vi "分层图显示1.2.1（看别的）.vi"(11 "IN":string) -> (3 "OUT":string)   [LabVIEW 2016]
uses:
  <vilib>/Utility/file.llb/Read Delimited Spreadsheet (DBL).vi
  <vilib>/Utility/file.llb/Read Delimited Spreadsheet (I64).vi
panel:
  in  "更换色码":bool
  in  "色码表导入":path=path "C:/Users/H301/Desktop/art闭环扫描程序/色码表/色码表（彩色2）.txt" caption="（色码表导入）"
  out "导入进度":u8(slide) scale=0.0..100.0
  in  "min":dbl format="%#_4e"
  in  "max":dbl format="%#_4e"
  in  "ESC":bool
  out "分层图":dbl[][](graph)
  in  "NEXT":bool
  in  "层数:":i32
  out "数组":dbl[][][](array[numeric])
  # "强度表"
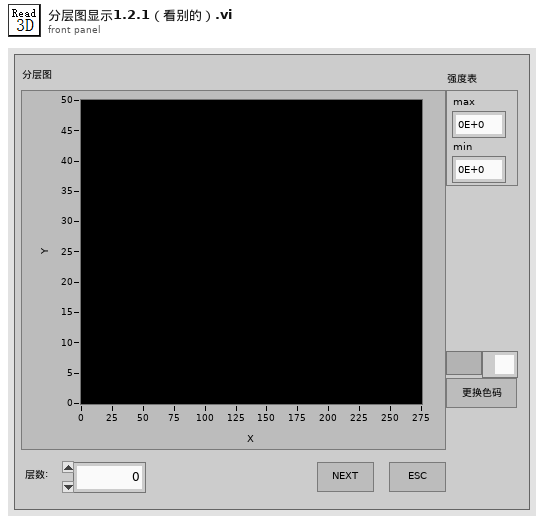
[diagram p1: front panel]
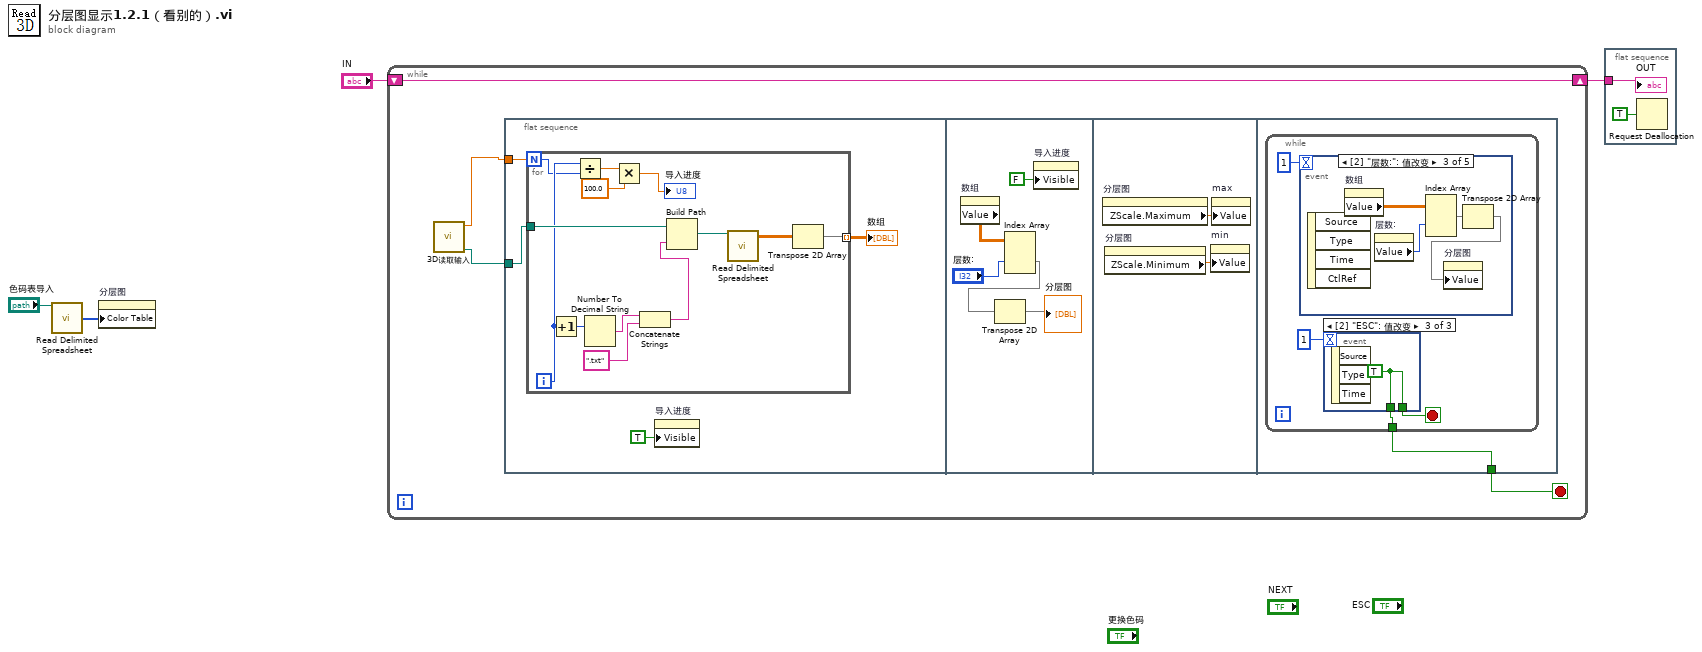
[diagram p0: block diagram]
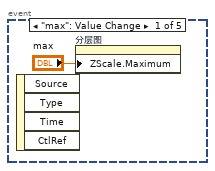
[diagram p2: hidden frame]
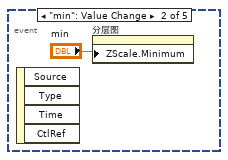
[diagram p3: hidden frame]
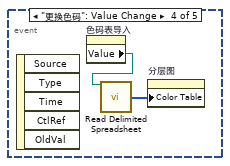
[diagram p4: hidden frame]
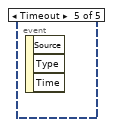
[diagram p5: hidden frame]
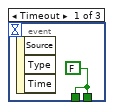
[diagram p6: hidden frame]
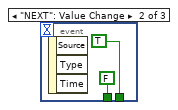
[diagram p7: hidden frame]
diagram:
  n1 = call-poly <vilib>:"Read Delimited Spreadsheet.vi"("file path (dialog if empty)"="色码表导入") -> ("first row"=w2:i64[])  [unwired: 9 in, 5 out]
  n2 = property on="分层图" class="IntGraph (严格)"("Color Table"=w2) -> ()  [unwired: 2 in, 2 out]
  n3 = while {
    shift-right: [w8] -> w3
    shift-left: "IN" -> [w8]
    stop <- w7 stop-if-true
    n4 = call "3D读取输入.vi"() -> ("文件读取路径"=w5:path, "行总数"=w6:dbl)  [unwired: 9 in, 1 out]
    n5 = flat-sequence {
      tunnel: w6 -> [w11]
      tunnel: w5 -> [w10]
      tunnel: [w33] -> w7
      frame #0 {
        n6 = for {
          N: w11 -> [w16]
          tunnel: [w24] -> w12 mode=indexing
          tunnel: w10 -> [w18]
          i -> [w17]
          n7 = Increment(x=w17) -> (x+1=w21:i32)
          n8 = Divide(x=w17, y=w16) -> (x/y=w15:dbl)
          n9 = Number To Decimal String(number=w21) -> (decimal integer string=w20:string)  [unwired: 1 in]
          n10 = Multiply(x=w15, y=100.0) -> (x*y=→"导入进度":dbl)
          n11 = Concatenate Strings(w20, ".txt") -> (w22:string)
          n12 = Build Path(base path=w18, name or relative path=w22) -> (appended path=w23:path)
          n13 = call-poly <vilib>:"Read Delimited Spreadsheet.vi"("file path (dialog if empty)"=w23) -> ("all rows"=w25:dbl[][])  [unwired: 9 in, 5 out]
          n14 = Transpose 2D Array(2D array=w25) -> (transposed array=w24:dbl[][])
        }
        "数组" <- w12
        n15 = property on="导入进度" class="Slide (严格)"("Visible"=TRUE ("可见")) -> ()  [unwired: 2 in, 2 out]
      }
      frame #1 {
        n16 = property on="数组" class="Arr (严格)"() -> ("Value"=w26:dbl[][][])  [unwired: 2 in, 2 out]
        n17 = Index Array(array=w26, index (dim 1)="层数:") -> (element=w28:dbl[][])  [unwired: 2 in]
        n18 = Transpose 2D Array(2D array=w28) -> (transposed array=→"分层图":dbl[][])
        n19 = property on="导入进度" class="Slide (严格)"("Visible"=FALSE ("可见")) -> ()  [unwired: 2 in, 2 out]
      }
      frame #2 {
        n20 = property on="分层图" class="IntGraph (严格)"() -> ("ZScale.Maximum"=w31:dbl)  [unwired: 2 in, 2 out]
        n21 = property on="分层图" class="IntGraph (严格)"() -> ("ZScale.Minimum"=w32:dbl)  [unwired: 2 in, 2 out]
        n22 = property on="min" class="DigNum (严格)"("Value"=w32) -> ()  [unwired: 2 in, 2 out]
        n23 = property on="max" class="DigNum (严格)"("Value"=w31) -> ()  [unwired: 2 in, 2 out]
      }
      frame #3 {
        n24 = while {
          tunnel: [w36] -> w33
          stop <- w37 stop-if-true
          n25 = event shown="[2] \"层数:\": 值改变" {
            selector: _ -> [_ _ _ _ _]
            dyn-events: _ -> [_ _ _ _ _]
            timeout: 1 -> [_ _ _ _ _]
            event "max": Value Change {
              n26 = event-data() -> ()  [unwired: 1 in, 4 out]
              n27 = property on="分层图" class="IntGraph (严格)"("ZScale.Maximum"="max") -> ()  [unwired: 2 in, 2 out]
            }
            event "min": Value Change {
              n28 = event-data() -> ()  [unwired: 1 in, 4 out]
              n29 = property on="分层图" class="IntGraph (严格)"("ZScale.Minimum"="min") -> ()  [unwired: 2 in, 2 out]
            }
            event "层数:": Value Change {
              n30 = event-data() -> ()  [unwired: 1 in, 4 out]
              n31 = property on="数组" class="Arr (严格)"() -> ("Value"=w40:dbl[][][])  [unwired: 2 in, 2 out]
              n32 = property on="层数:" class="DigNum (严格)"() -> ("Value"=w43:i32)  [unwired: 2 in, 2 out]
              n33 = Index Array(array=w40, index (dim 1)=w43) -> (element=w42:dbl[][])  [unwired: 2 in]
              n34 = Transpose 2D Array(2D array=w42) -> (transposed array=w41:dbl[][])
              n35 = property on="分层图" class="IntGraph (严格)"("Value"=w41) -> ()  [unwired: 2 in, 2 out]
            }
            event "更换色码": Value Change {
              n36 = event-data() -> ()  [unwired: 1 in, 5 out]
              n37 = property on="色码表导入" class="Path"() -> ("Value"=w44:path)  [unwired: 2 in, 2 out]
              n38 = call-poly <vilib>:"Read Delimited Spreadsheet.vi"("file path (dialog if empty)"=w44) -> ("first row"=w45:i64[])  [unwired: 9 in, 5 out]
              n39 = property on="分层图" class="IntGraph (严格)"("Color Table"=w45) -> ()  [unwired: 2 in, 2 out]
            }
            event Timeout {
              n40 = event-data() -> ()  [unwired: 1 in, 3 out]
            }
          }
          n41 = event shown="[2] \"ESC\": 值改变" {
            selector: _ -> [_ _ _]
            dyn-events: _ -> [_ _ _]
            timeout: 1 -> [_ _ _]
            tunnel: [w46 TRUE w49] -> w37
            tunnel: [w46 FALSE w49] -> w36
            event Timeout {
              w46 = FALSE
              n42 = event-data() -> ()  [unwired: 1 in, 3 out]
            }
            event "NEXT": Value Change {
              n43 = event-data() -> ()  [unwired: 1 in, 3 out]
            }
            event "ESC": Value Change {
              w49 = TRUE
              n44 = event-data() -> ()  [unwired: 1 in, 3 out]
            }
          }
        }
      }
    }
  }
  n45 = flat-sequence {
    tunnel: w3 -> [w51]
    frame #0 {
      n46 = Request Deallocation(TRUE ("标志")) -> ()
      "OUT" <- w51
    }
  }
